vi "Tracking_SubVI-4.vi"(7 "[IN] Control Parameters":T4, 8 "error IN":errorcluster, 9 "[IN] Before-After Tracks":T3, 11 "[IN] Movie Values":T2 {"Particle Fil Setups"."Type of particle filter"."Measurement Parameter" items=["Center of Mass X", "Center of Mass Y", "First Pixel X", "First Pixel Y", "Bounding Rect Left", "Bounding Rect Top", "Bounding Rect Right", "Bounding Rect Bottom", "Max Feret Diameter Start X", "Max Feret Diameter Start Y", "Max Feret Diameter End X", "Max Feret Diameter End Y", "Max Horiz. Segment Length Left", "Max Horiz. Segment Length Right", "Max Horiz. Segment Length Row", "-", "Bounding Rect Width", "Bounding Rect Height", "Bounding Rect Diagonal", "Perimeter", "Convex Hull Perimeter", "Holes' Perimeter", "Max Feret Diameter", "Equivalent Ellipse Major Axis", "Equivalent Ellipse Minor Axis", "Equivalent Ellipse Minor Axis (Feret)", "Equivalent Rect Long Side", "Equivalent Rect Short Side", "Equivalent Rect Diagonal", "Equivalent Rect Short Side (Feret)", "Average Horiz. Segment Length", "Average Vert. Segment Length", "Hydraulic Radius", "Waddel Disk Diameter", "-", "Area", "Holes' Area", "Particle & Holes' Area", "Convex Hull Area", "Image Area", "-", "Number of Holes", "Number of Horiz. Segments", "Number of Vert. Segments", "-", "Orientation", "Max Feret Diameter Orientation", "-", "% Area/Image Area", "% Area/(Particle & Holes' Area)", "Ratio of Equivalent Ellipse Axes", "Ratio of Equivalent Rect Sides", "-", "Elongation Factor", "Compactness Factor", "Heywood Circularity Factor", "Type Factor", "-", "Sum X", "Sum Y", "Sum XX", "Sum XY", "Sum YY", "Sum XXX", "Sum XXY", "Sum XYY", "Sum YYY", "-", "Moment of Inertia XX", "Moment of Inertia XY", "Moment of Inertia YY", "Moment of Inertia XXX", "Moment of Inertia XXY", "Moment of Inertia XYY", "Moment of Inertia YYY", "Norm. Moment of Inertia XX", "Norm. Moment of Inertia XY", "Norm. Moment of Inertia YY", "Norm. Moment of Inertia XXX", "Norm. Moment of Inertia XXY", "Norm. Moment of Inertia XYY", "Norm. Moment of Inertia YYY", "Hu Moment 1", "Hu Moment 2", "Hu Moment 3", "Hu Moment 4", "Hu Moment 5", "Hu Moment 6", "Hu Moment 7"]}) -> (0 "error OUT":errorcluster, 1 "[OUT] Before-After Tracks":T3, 3 "[OUT] Obtained Movie Values":T2 {"Particle Fil Setups"."Type of particle filter"."Measurement Parameter" items=["Center of Mass X", "Center of Mass Y", "First Pixel X", "First Pixel Y", "Bounding Rect Left", "Bounding Rect Top", "Bounding Rect Right", "Bounding Rect Bottom", "Max Feret Diameter Start X", "Max Feret Diameter Start Y", "Max Feret Diameter End X", "Max Feret Diameter End Y", "Max Horiz. Segment Length Left", "Max Horiz. Segment Length Right", "Max Horiz. Segment Length Row", "-", "Bounding Rect Width", "Bounding Rect Height", "Bounding Rect Diagonal", "Perimeter", "Convex Hull Perimeter", "Holes' Perimeter", "Max Feret Diameter", "Equivalent Ellipse Major Axis", "Equivalent Ellipse Minor Axis", "Equivalent Ellipse Minor Axis (Feret)", "Equivalent Rect Long Side", "Equivalent Rect Short Side", "Equivalent Rect Diagonal", "Equivalent Rect Short Side (Feret)", "Average Horiz. Segment Length", "Average Vert. Segment Length", "Hydraulic Radius", "Waddel Disk Diameter", "-", "Area", "Holes' Area", "Particle & Holes' Area", "Convex Hull Area", "Image Area", "-", "Number of Holes", "Number of Horiz. Segments", "Number of Vert. Segments", "-", "Orientation", "Max Feret Diameter Orientation", "-", "% Area/Image Area", "% Area/(Particle & Holes' Area)", "Ratio of Equivalent Ellipse Axes", "Ratio of Equivalent Rect Sides", "-", "Elongation Factor", "Compactness Factor", "Heywood Circularity Factor", "Type Factor", "-", "Sum X", "Sum Y", "Sum XX", "Sum XY", "Sum YY", "Sum XXX", "Sum XXY", "Sum XYY", "Sum YYY", "-", "Moment of Inertia XX", "Moment of Inertia XY", "Moment of Inertia YY", "Moment of Inertia XXX", "Moment of Inertia XXY", "Moment of Inertia XYY", "Moment of Inertia YYY", "Norm. Moment of Inertia XX", "Norm. Moment of Inertia XY", "Norm. Moment of Inertia YY", "Norm. Moment of Inertia XXX", "Norm. Moment of Inertia XXY", "Norm. Moment of Inertia XYY", "Norm. Moment of Inertia YYY", "Hu Moment 1", "Hu Moment 2", "Hu Moment 3", "Hu Moment 4", "Hu Moment 5", "Hu Moment 6", "Hu Moment 7"]}, 4 "[OUT] Number of \nRaw Displacements":i32)   [LabVIEW 2013]
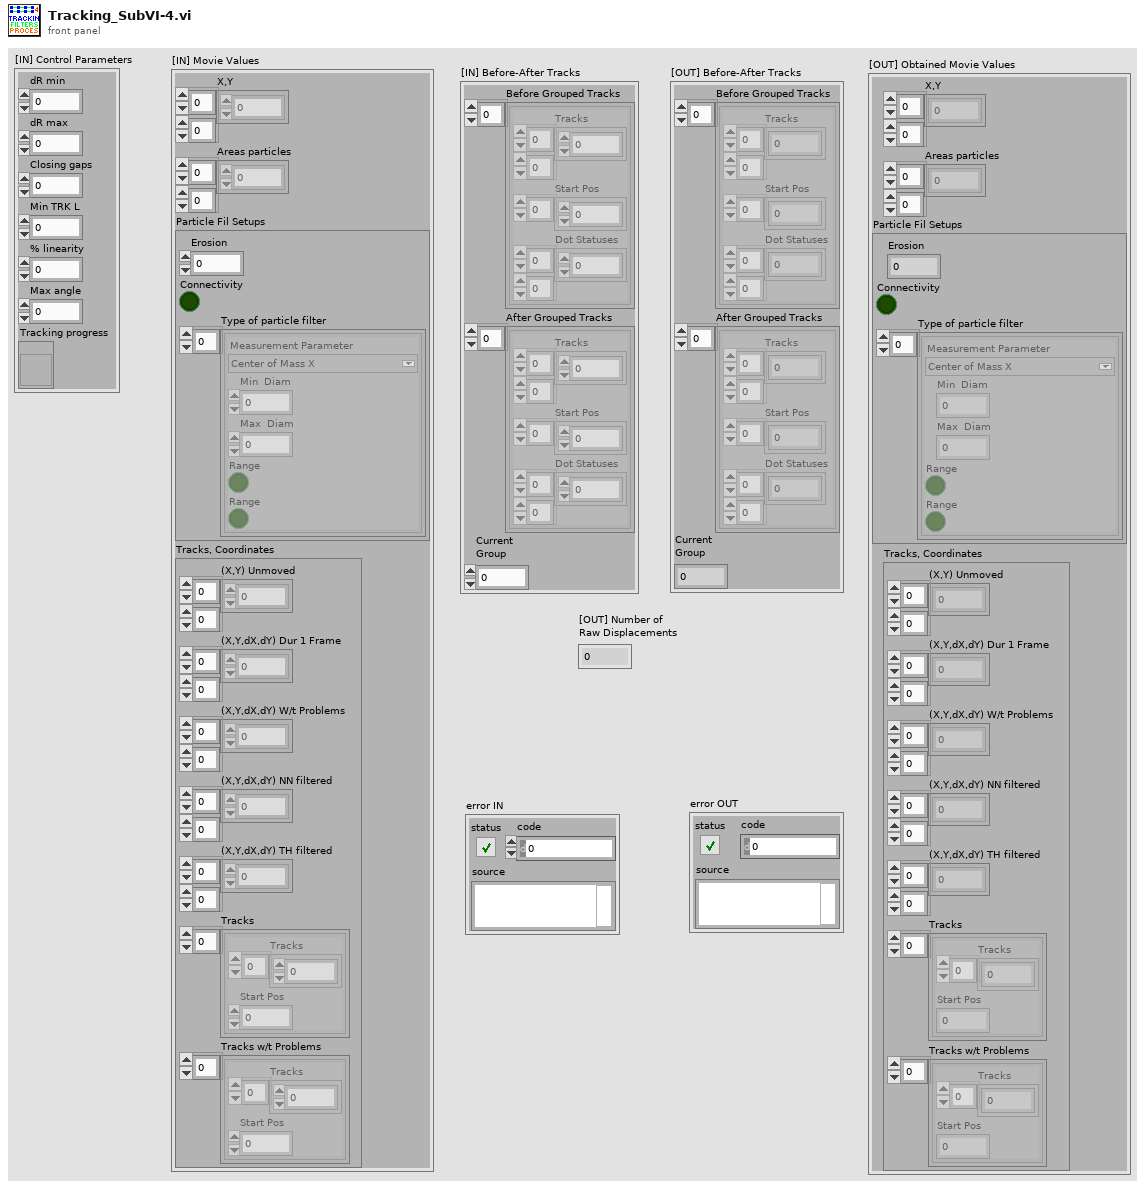
[diagram p1: front panel]
types:
  T1 = typedef "Particle Parameters" = i32
  T2 = cluster{"X,Y":dbl[][], "Areas particles":dbl[][], "Particle Fil Setups":cluster{"Erosion":i32, "Connectivity ":bool, "Type of particle filter":cluster{"Measurement Parameter":T1, "Min  Diam":dbl, "Max  Diam":dbl, "Range":bool, "Range":bool}[]}, "Tracks, Coordinates":cluster{"(X,Y) Unmoved":dbl[][], "(X,Y,dX,dY) Dur 1 Frame":dbl[][], "(X,Y,dX,dY) W/t Problems":dbl[][], "(X,Y,dX,dY) NN filtered":dbl[][], "(X,Y,dX,dY) TH filtered":dbl[][], "Tracks":cluster{"Tracks":dbl[], "Start Pos":i32}[], "Tracks w/t Problems":cluster{"Tracks":dbl[], "Start Pos":i32}[]}}
  T3 = cluster{"Before Grouped Tracks":cluster{"Tracks":dbl[][], "Start Pos":i32[], "Dot Statuses":i16[][]}[], "After Grouped Tracks":cluster{"Tracks":dbl[][], "Start Pos":i32[], "Dot Statuses":i16[][]}[], "Current\nGroup":i32}
  T4 = cluster{"dR min ":dbl, "dR max ":dbl, "Closing gaps":i32, "Min TRK L":i32, "% linearity":i32, "Max angle":dbl, "Tracking progress":refnum<vi>}
  T5 = cluster{"X,Y":dbl[][], "Areas particles":dbl[][], "Particle Fil Setups":cluster{"Erosion":i32, "Connectivity ":bool, "Type of particle filter":cluster{"Measurement Parameter":T1, "Min  Diam":dbl, "Max  Diam":dbl, "Range":bool, "Range":bool}[]}, "Tracks, Coordinates":cluster{"(X,Y) Unmoved":dbl[][], "(X,Y,dX,dY) Dur 1 Frame":dbl[][], "(X,Y,dX,dY) whole (dt>1)":dbl[][], "(X,Y,dX,dY) NN filtered":dbl[][], "(X,Y,dX,dY) TH filtered":dbl[][], "Tracks + Starting Position":cluster{"Tracks":dbl[], "Start Pos":i32}[]}}
  T6 = cluster{"Erosion":i32, "Connectivity ":bool, "Type of particle filter":cluster{"Measurement Parameter":T1, "Min  Diam":dbl, "Max  Diam":dbl, "Range":bool, "Range":bool}[]}
  T7 = cluster{"(X,Y) Unmoved":dbl[][], "(X,Y,dX,dY) Dur 1 Frame":dbl[][], "(X,Y,dX,dY) W/t Problems":dbl[][], "(X,Y,dX,dY) NN filtered":dbl[][], "(X,Y,dX,dY) TH filtered":dbl[][], "Tracks":cluster{"Tracks":dbl[], "Start Pos":i32}[], "Tracks w/t Problems":cluster{"Tracks":dbl[], "Start Pos":i32}[]}
  T8 = cluster{"Tracks W/T Problems":dbl[], "Start Pos":i32}[]
  T9 = cluster{"Tracks":dbl[][], "Start Pos":i32[], "Dot Statuses":i16[][]}[]
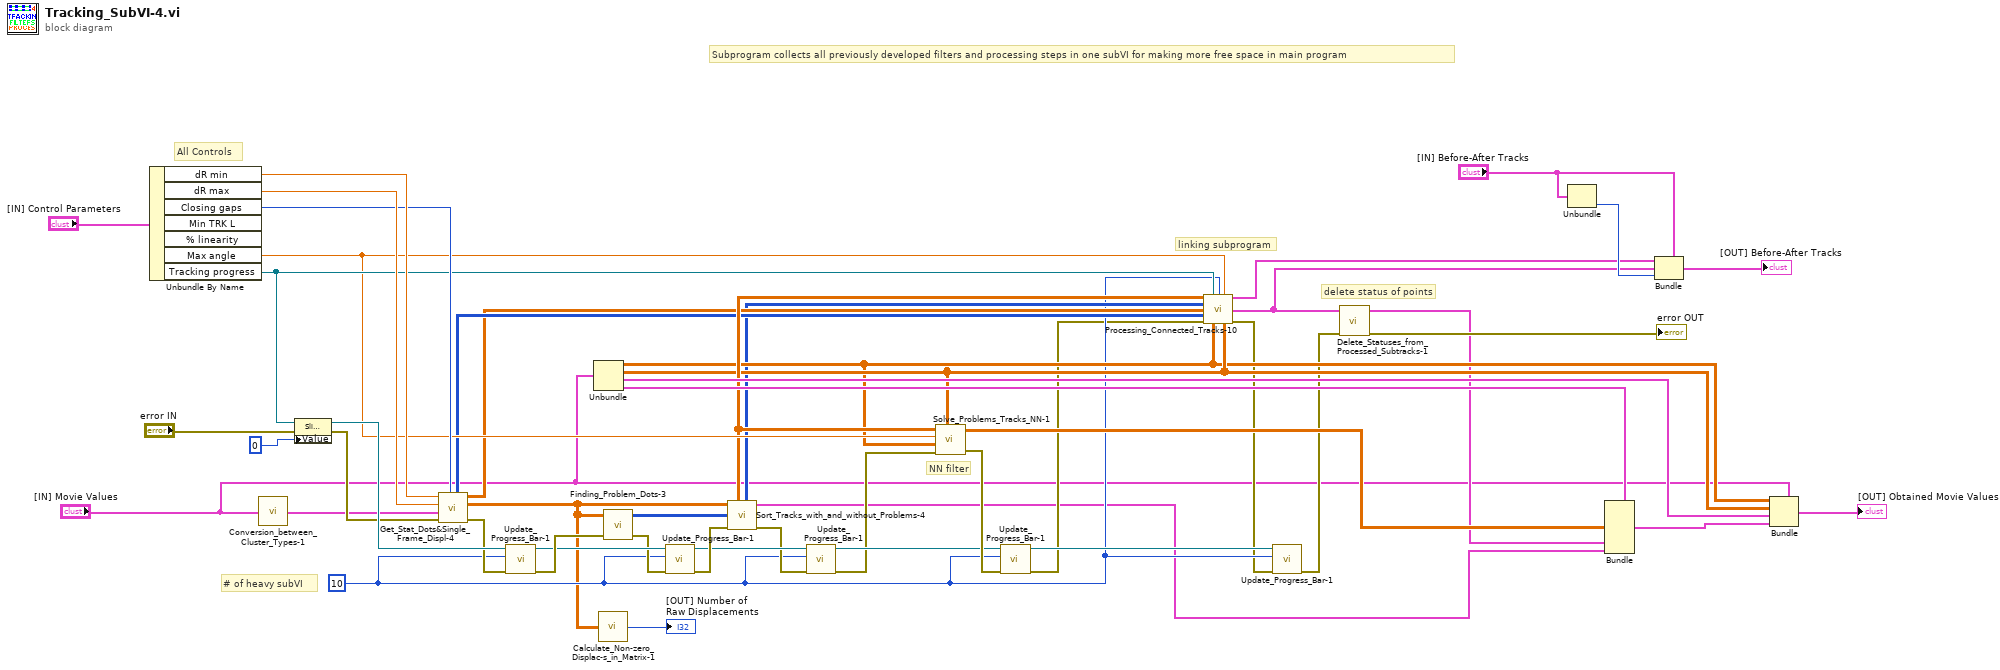
[diagram p0: block diagram]
diagram:
  w14 = 10 ("[IN] Number of SubVI")
  # "linking subprogram"
  # "delete status of points"
  # "Subprogram collects all previously developed filters and processing steps in one subVI for making more free space in main program"
  # "NN filter"
  # "# of heavy subVI"
  # "All Controls"
  n1 = Unbundle By Name("[IN] Control Parameters") -> ("dR min"=w31:dbl, "dR max"=w30:dbl, "Closing gaps"=w28:i32, "Max angle"=w25:dbl, "Tracking progress"=w26:refnum<vi>)  [unwired: 2 out]
  n2 = call "Conversion_between_Cluster_Types-1.vi"("[IN] New Movie Values"="[IN] Movie Values") -> ("[OUT] Old Movie Values"=w4:T5)
  n3 = property on="Property Node" class="Slide (strict)"(reference=w26, error in="error IN", "Value"=u8 0) -> (reference out=w33:refnum<vi>, error out=w29:errorcluster)
  n4 = call "Get_Stat_Dots&Single_Frame_Displ-4.vi"("Closing gaps"=w28, "[IN] error"=w29, "[IN] Movie Values"=w4, "dR max"=w30, "dR min"=w31) -> ("error OUT"=w27:errorcluster, "[OUT] Displacements \nwith Length >1 Frame"=w2:dbl[][], "[OUT] (X,Y) Poten-\ntially Moving"=w18:dbl[][], "[OUT] Dot matrix after using \nsome filters which contains \ndots with increased statuses"=w19:i16[][])  [unwired: 3 out]
  n5 = call "Update_Progress_Bar-1.vi"("error IN"=w27, "[IN] Number of SubVI"=w14, "[IN] Tracking progress"=w33) -> ("error OUT"=w47:errorcluster, "[OUT] Tracking progress"=w46:refnum<vi>)  [unwired: 3 in]
  n6 = Unbundle("[IN] Movie Values") -> ("X,Y"=w20:dbl[][], "Areas particles"=w21:dbl[][], "Particle Fil Setups"=w41:T6, "Tracks, Coordinates"=w40:T7)
  n7 = call "Calculate_Non-zero_Displac-s_in_Matrix-1.vi"("[IN] Displacements \nFrm-to-Frm In Cols"=w2) -> ("[OUT] Number of \n(X,Y,dX,dY) displ-s"=→"[OUT] Number of \nRaw Displacements":i32)
  n8 = call "Finding_Problem_Dots-3.vi"("error IN"=w47, "[IN] Frame-to-frame displ"=w2) -> ("error OUT"=w45:errorcluster, "[OUT] Dot matrix"=w48:i16[][])  [unwired: 2 in]
  n9 = call "Update_Progress_Bar-1.vi"("error IN"=w45, "[IN] Number of SubVI"=w14, "[IN] Tracking progress"=w46) -> ("error OUT"=w44:errorcluster, "[OUT] Tracking progress"=w43:refnum<vi>)  [unwired: 3 in]
  n10 = call "Sort_Tracks_with_and_without_Problems-4.vi"("error IN"=w44, "[IN] Dot matrix"=w48, "[IN}Frame-to-frame displ"=w2) -> ("error OUT"=w42:errorcluster, "[OUT] Tracks w/t Problems"=w6:T8, "[OUT] Filtered Dot Matrix"=w17:i16[][], "[OUT] Displacements with problems\nCollected in Columns (as raw displ)"=w24:dbl[][])  [unwired: 2 in, 1 out]
  n11 = call "Update_Progress_Bar-1.vi"("error IN"=w42, "[IN] Number of SubVI"=w14, "[IN] Tracking progress"=w43) -> ("error OUT"=w9:errorcluster, "[OUT] Tracking progress"=w10:refnum<vi>)  [unwired: 3 in]
  n12 = call "Solve_Problems_Tracks_NN-1.vi"("Tracks (unsorted, cols)"=w24, "Max angle"=w25, "X,Y"=w20, "error IN"=w9, "Areas"=w21) -> ("Tracks (X,Y,dX,dY)"=w16:dbl[][], "error OUT"=w38:errorcluster)  [unwired: 1 out]
  n13 = call "Update_Progress_Bar-1.vi"("error IN"=w38, "[IN] Number of SubVI"=w14, "[IN] Tracking progress"=w10) -> ("error OUT"=w13:errorcluster, "[OUT] Tracking progress"=w15:refnum<vi>)  [unwired: 3 in]
  n14 = call "Processing_Connected_Tracks-10.vi"("[IN] Unsorted \nProblem Tracks"=w24, "[IN] Tracking progress"=w26, "[IN] Number of SubVI"=w14, "[IN] Max angle"=w25, "[IN] Dot matrix \nfor moving points\n(splitted tracks)"=w17, "[IN] Potentially\nMoving (X,Y)"=w18, "[IN] Dot matrix with \nstatuses for potentially \nmoving dots"=w19, "error IN"=w13, "[IN] Primary \n(X,Y) Detected"=w20, "[IN] Areas particles\nPrimary Detected"=w21) -> ("[OUT] Before Processing Tracks"=w23:T9, "[OUT] Processed Tracks"=w22:T9, "error OUT"=w12:errorcluster)  [unwired: 3 in]
  n15 = call "Update_Progress_Bar-1.vi"("error IN"=w12, "[IN] Number of SubVI"=w14, "[IN] Tracking progress"=w15) -> ("error OUT"=w11:errorcluster)  [unwired: 3 in, 1 out]
  n16 = call "Delete_Statuses_from_Processed_Subtracks-1.vi"("error IN"=w11, "[IN] Processed Tracks"=w22) -> ("error OUT"=→"error OUT":errorcluster, "[OUT] Tracks"=w7:cluster{"Track":dbl[], "Start Pos":i32}[])  [unwired: 4 in]
  n17 = Unbundle("[IN] Before-After Tracks") -> ("Current\nGroup"=w36:i32)  [unwired: 2 out]
  n18 = Bundle(cluster=w40, "(X,Y,dX,dY) NN filtered"=w16, "Tracks"=w7, "Tracks w/t Problems"=w6) -> (w39:T7)  [unwired: 4 in]
  n19 = Bundle(cluster="[IN] Before-After Tracks", "Before Grouped Tracks"=w23, "After Grouped Tracks"=w22, "Current\nGroup"=w36) -> (→"[OUT] Before-After Tracks":T3)
  n20 = Bundle(cluster="[IN] Movie Values", "X,Y"=w20, "Areas particles"=w21, "Particle Fil Setups"=w41, "Tracks, Coordinates"=w39) -> (→"[OUT] Obtained Movie Values":T2)
